vi "Hash String with SHA-256.vi"(8 "error_n":errorcluster, 11 "string":string) -> (0 "error_out":errorcluster, 3 "hash":string)   [LabVIEW 2019]
doc: "Calculate a SHA-256 cryptogrpahic hash for a given input string.\n\nImplements the SHA-2 256 encryption algorithm (approximately as described by the wikipedia page pseudocode)."
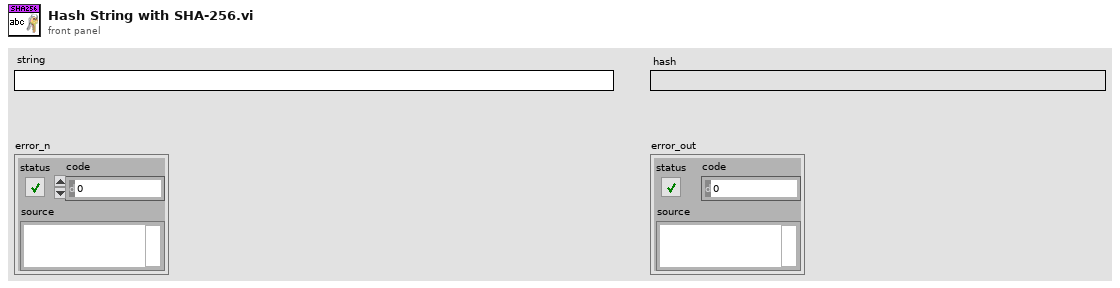
[diagram p1: front panel]
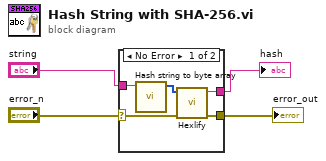
[diagram p0: block diagram]
diagram:
  n1 = case shown="No Error" "error_n" {
    selector: "error_n" -> [w5 w10]
    tunnel: "string" -> [w9 _]
    tunnel: [w7 _] -> w1
    tunnel: [w6 w10] -> w3
    frame No Error {
      n2 = call "Hash string to byte array.vi"("String to Encode"=w9) -> ("H Array"=w8:u32[])  [unwired: 10 in]
      n3 = call "Hexlify.vi"("error in (no error)"=w5, "H Array"=w8) -> ("error out"=w6:errorcluster, "String"=w7:string)  [unwired: 8 in]
    }
    frame Error {
    }
  }
  "hash" <- w1
  "error_out" <- w3
